vi "Review ROCs Dialog.vi"(8 "error in (no error)":errorcluster) -> (0 "error out":errorcluster, 2 "Canceled":bool)   [LabVIEW 2011]
panel:
  in  "OK Button":bool
  in  "Cancel Button":bool
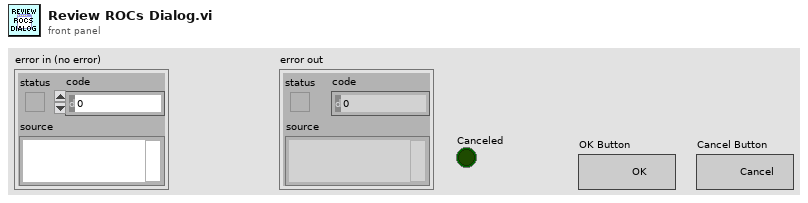
[diagram p1: front panel]
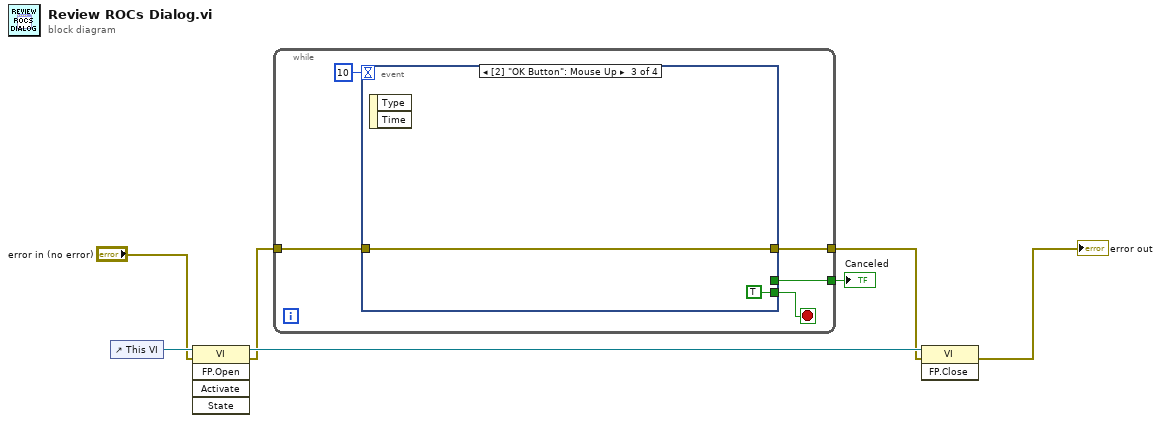
[diagram p0: block diagram]
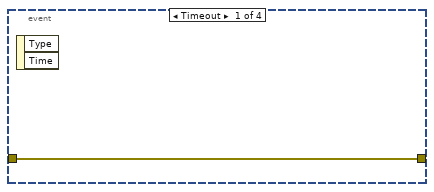
[diagram p2: hidden frame]
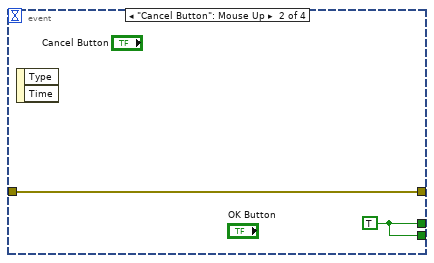
[diagram p3: hidden frame]
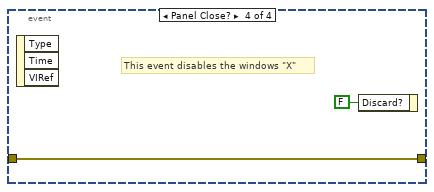
[diagram p4: hidden frame]
diagram:
  n1 = control-ref of="This VI"() -> (w7:refnum<vi>)
  n2 = invoke class="VI" method="FP.Open"(reference=w7, error in="error in (no error)") -> (reference out=w6:refnum<vi>, error out=w2:errorcluster)  [unwired: 3 in, 3 out]
  n3 = while {
    tunnel: [w8] -> w3
    tunnel: w2 -> [w9]
    tunnel: [w10] -> w1
    stop <- w11 stop-if-true
    n4 = event shown="[2] \"OK Button\": Mouse Up" {
      selector: _ -> [_ _ _ _]
      dyn-events: _ -> [_ _ _ _]
      timeout: 10 -> [_ _ _ _]
      tunnel: [_ w14 TRUE _] -> w11
      tunnel: [w13 w15 w17 w18] -> w10
      tunnel: w9 -> [w13 w15 w17 w18]
      tunnel: [_ w14 _ _] -> w8
      event Timeout {
        n5 = event-data() -> ()  [unwired: 1 in, 2 out]
      }
      event "Cancel Button": Mouse Up {
        w14 = TRUE
        n6 = event-data() -> ()  [unwired: 1 in, 2 out]
      }
      event "OK Button": Mouse Up {
        n7 = event-data() -> ()  [unwired: 1 in, 2 out]
      }
      event Panel Close? {
        # "This event disables the windows \"X\""
        n8 = event-data() -> ()  [unwired: 1 in, 3 out]
        n9 = event-data("Discard?"=FALSE) -> ()  [unwired: 1 in, 1 out]
      }
    }
  }
  "Canceled" <- w3
  n10 = invoke class="VI" method="FP.Close"(reference=w6, error in=w1) -> (error out=→"error out":errorcluster)  [unwired: 1 in, 2 out]
